vi "Fetch&Process_Measurements.vi"(7 "Rolling Timer Input":timestamp, 8 "error in (no error)":errorcluster, 9 "Initial Time":timestamp, 10 "DCPowerInformation_byChannel":T1(array[cluster]), 11 "Queue Data Parameters in":T2) -> (0 "error out":errorcluster, 1 "Current Measurement":waveform(dbl)[](array[waveform]), 2 "Voltage Measurement":waveform(dbl)[](array[waveform]), 3 "Queue Data Parameters out":T2, 5 "Rolling Timer Output":timestamp)   [LabVIEW 2019]
uses:
  Controls/QueueDataControl.ctl
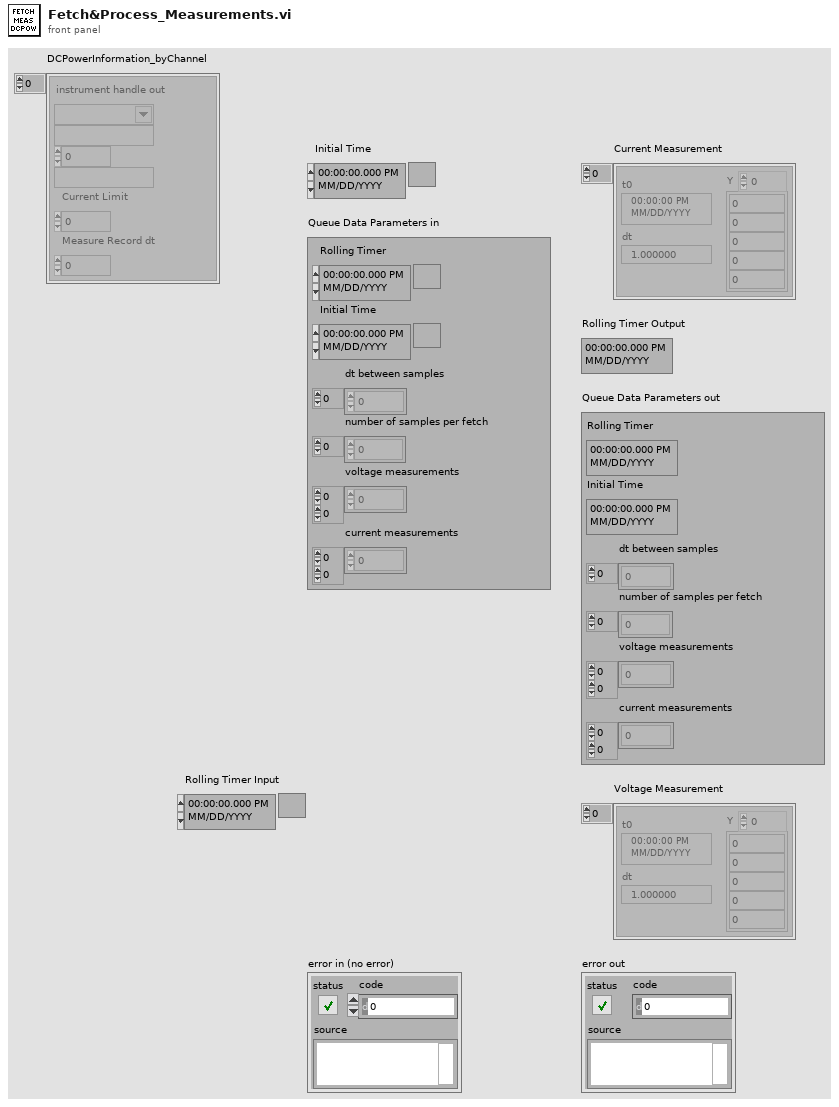
[diagram p1: front panel]
types:
  T1 = cluster{"instrument handle out":refnum<k15>, string, dbl, string, "Current Limit":dbl, "Measure Record dt":dbl}[]
  T2 = typedef "QueueDataControl.ctl" = cluster{"Rolling Timer":timestamp, "Initial Time":timestamp, "dt between samples":dbl[], "number of samples per fetch":i32[], "voltage measurements":dbl[][], "current measurements":dbl[][]}
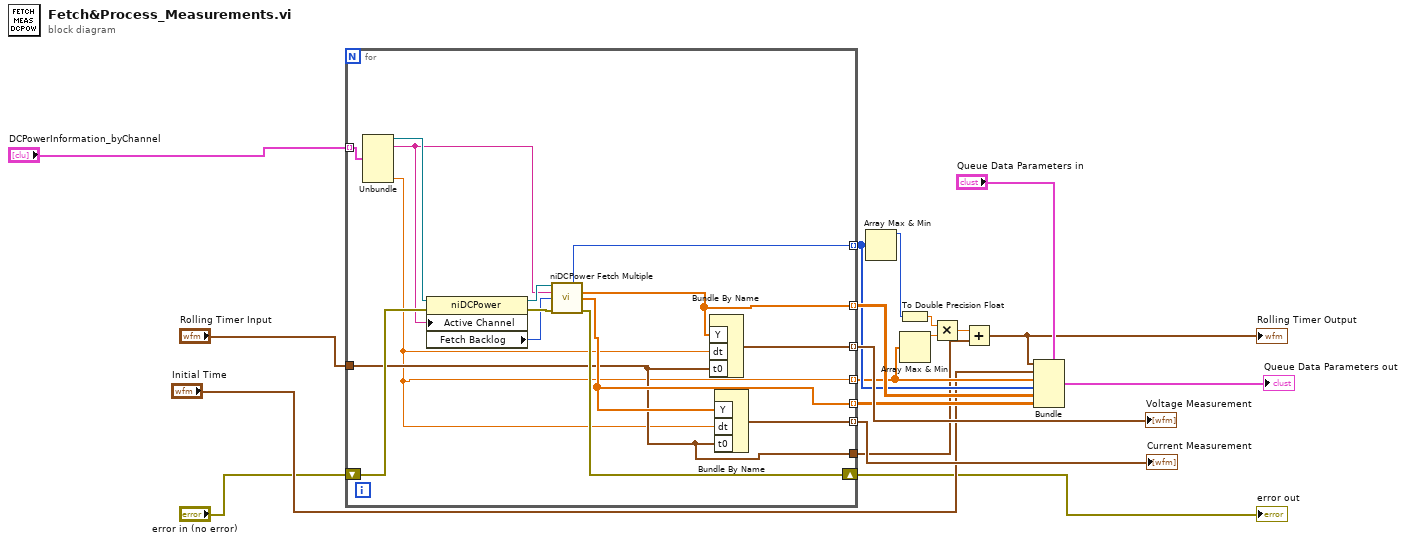
[diagram p0: block diagram]
diagram:
  n1 = for {
    tunnel: "DCPowerInformation_byChannel" -> [w34] mode=indexing
    shift-right: [w29] -> w3
    shift-left: "error in (no error)" -> [w33]
    tunnel: "Rolling Timer Input" -> [w21]
    tunnel: [w26] -> w16 mode=indexing
    tunnel: [w25] -> w17 mode=indexing
    tunnel: [w24] -> w13 mode=indexing
    tunnel: [w23] -> w14 mode=indexing
    tunnel: [w22] -> w15 mode=indexing
    tunnel: [w20] -> w12 mode=indexing
    tunnel: [w21] -> w9
    n2 = Unbundle(w34) -> ("instrument handle out"=w31:refnum<k15>, w27:string, "Measure Record dt"=w20:dbl)  [unwired: 3 out]
    n3 = property class="niDCPower"(reference=w31, error in=w33, "Active Channel"=w27) -> (reference out=w30:refnum<k15>, error out=w32:errorcluster, "Fetch Backlog"=w28:i32)
    n4 = call <instrlib>:"niDCPower Fetch Multiple.vi"("instrument handle"=w30, "channel name"=w27, "count (1)"=w28, "error in (no error)"=w32) -> ("actual count"=w24:i32, "voltage measurements"=w23:dbl[], "current measurements"=w22:dbl[], "error out"=w29:errorcluster)  [unwired: 6 in, 2 out]
    n5 = Bundle By Name("Y"=w23, "dt"=w20, "t0"=w21) -> (w26:waveform(dbl))  [unwired: 1 out]
    n6 = Bundle By Name("Y"=w22, "dt"=w20, "t0"=w21) -> (w25:waveform(dbl))  [unwired: 1 out]
  }
  "Current Measurement" <- w17
  "Voltage Measurement" <- w16
  "error out" <- w3
  n7 = Array Max & Min(array=w13) -> (max value=w5:i32)  [unwired: 3 out]
  n8 = To Double Precision Float(number=w5) -> (double precision float=w6:dbl)
  n9 = Array Max & Min(array=w12) -> (max value=w7:dbl)  [unwired: 3 out]
  n10 = Multiply(x=w6, y=w7) -> (x*y=w8:dbl)
  n11 = Add(x=w8, y=w9) -> (x+y=w10:timestamp)
  "Rolling Timer Output" <- w10
  n12 = Bundle(cluster="Queue Data Parameters in", "Rolling Timer"=w10, "Initial Time"="Initial Time", "dt between samples"=w12, "number of samples per fetch"=w13, "voltage measurements"=w14, "current measurements"=w15) -> (→"Queue Data Parameters out":T2)
